vi "Array - Not Empty.vi"() -> ()   [LabVIEW 2017, in "Assertions.Tests.lvlib" / "Assert Collection Empty.lvlib"]
uses:
  Assert Collection Empty.lvlib
  cbee6d11-a8dd-48ad-99e8-9ee3396d33d5.vi
  src/Transparent Assertions/Constraints/Collection Is Empty/Collection Is Empty.lvclass
  src/Transparent Assertions/Assertions/Assertions.lvlib
panel:
  out "error out":errorcluster
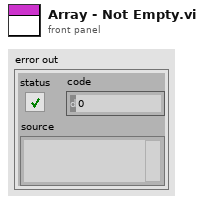
[diagram p1: front panel]
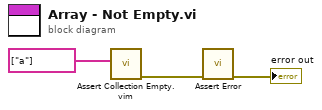
[diagram p0: block diagram]
diagram:
  n1 = call "Assert Collection Empty.vim"("Collection"=string[] ["a"]) -> ("error out"=w2:errorcluster)  [unwired: 10 in]
  n2 = call "Assert Error.vi"("error in (no error)"=w2) -> ("error out"=→"error out":errorcluster)  [unwired: 10 in]
